vi "SYST_PRES.vi"(0 "VISA IN":refnum<visa-resource-name>, 5 "error in":errorcluster) -> (14 "VISA Out":refnum<visa-resource-name>, 19 "error out":errorcluster)   [LabVIEW 2018, in "PNA-X.lvlib"] (continued)
\n(Read-Write) Sets the type of the specified marker. \nSee Critical Note \nParameters \n<cnum> Channel number of the measurement. There must be a selected measurement \non that channel. If unspecified, <cnum> is set to 1. \n<mkr> Any marker number from 1 to 10; if unspecified, value is set to 1 \n<char> Choose from: \nNORMal - a marker that stays on the assigned X-axis position unless moved or \nsearching. \nFIXed - a marker that will not leave the assigned X or current Y-axis position. \nExamples CALC:MARK:TYPE NORM \ncalculate2:marker2:type fixed \nQuery Syntax CALCulate<cnum>:MARKer<mkr>:TYPE? \nReturn Type Character \n1540\n\nDefault NORMal \nCALCulate<cnum>:MARKer<mkr>:SET <char> \n(Write-only) Sets the selected instrument setting to assume the value of the specified marker. \nMarker Functions CENT, SPAN, STARt, and STOP do not work with channels that are in CW or \nSegment Sweep mode. \nSee Critical Note \nParameters \n<cnum> Channel number of the measurement. There must be a selected measurement \non that channel. If unspecified, <cnum> is set to 1. \n<mkr> Any marker number from 1 to 10; if unspecified, value is set to 1 \n<char> Choose from: \nCENTer - changes center frequency to the value of the marker \nSPAN - changes the sweep span to the span that is defined by the delta marker \nand the marker that it references. Unavailable if there is no delta marker. \nSTARt - changes the start frequency to the value of the marker \nSTOP - changes the stop frequency to the value of the marker \nRLEVel - changes the reference level to the value of the marker \nDELay - changes the line length at the receiver input to the phase slope at the \nactive marker stimulus position. \nExamples CALC:MARK:SET CENT \ncalculate2:marker8:set span \nQuery Syntax Not Applicable \nDefault Not Applicable \nCALCulate<cnum>:MARKer<mkr>[:STATe] <ON|OFF> \n1541\n\n(Read-Write) Turns the specified marker ON or OFF. Marker 10 is the Reference Marker. To turn \nall markers off, use CALC:MARK:AOFF. \nSee Critical Note \nParameters \n<cnum> Channel number of the measurement. There must be a selected measurement \non that channel. If unspecified, <cnum> is set to 1. \n<mkr> Any marker number from 1 to 10; if unspecified, value is set to 1. \n<ON|OFF> ON (or 1) - turns marker ON. \nOFF (or 0) - turns marker OFF. \nExamples CALC:MARK ON \ncalculate2:marker8 on \nQuery Syntax CALCulate<cnum>:MARKer<mkr>:STATe? \nReturn Type Boolean (1 = ON, 0 = OFF) \nDefault Off \nCALCulate<cnum>:MARKer<mkr>:X <num> \n(Read-Write) Sets the marker's X-axis value (frequency, power, or time). If the marker is set as delta, \nthe SET and QUERY data is relative to the reference marker. \nSee Critical Note \nParameters \n<cnum> Channel number of the measurement. There must be a selected measurement \non that channel. If unspecified, <cnum> is set to 1. \n<mkr> Any marker number from 1 to 10; if unspecified, value is set to 1. \n<num> Any X-axis position within the measurement span of the marker. \nNote: This command will accept MIN or MAX instead of a numeric \nparameter. See SCPI Syntax for more information. \nExamples CALC:MARK:X 100Mhz \ncalculate2:marker8:x maximum \nQuery Syntax CALCulate<cnum>:MARKer<mkr>:X? \nReturn Type Numeric \nDefault First Marker turns ON in the middle of the X-axis span. Subsequent markers \nturn ON at the position of the active marker. \n1542\n\nCALCulate<cnum>:MARKer<mkr>:Y? \n(Read-only) Reads the marker's Y-axis value. The format of the value depends on the current \nCALC:MARKER:FORMAT setting. If the marker is set as delta, the data is relative to the reference \nmarker. The query always returns two numbers: \nSmith and Polar formats - (Real, Imaginary) \nLINPhase and LOGPhase - (Real, Imaginary) \nAll other formats - (Value,0) \nNote: To accurately read the marker Y-axis value with trace smoothing applied, the requested format \nmust match the displayed format. Otherwise, the returned value is un-smoothed data. For example, to \nread the smoothed marker value when measuring group delay, both the display format and the marker \nformat must be set to (Group) Delay. \nSee Critical Note \nParameters \n<cnum> Channel number of the measurement. There must be a selected measurement \non that channel. If unspecified, <cnum> is set to 1. \n<mkr> Any marker number from 1 to 10; if unspecified, value is set to 1. \nExamples CALC:MARK:Y? \ncalculate2:marker3:y? \nQuery Syntax CALCulate<cnum>:MARKer<mkr>:Y? \nReturn Type Numeric \nDefault Not applicable \nLast modified: \nMarch 27, 2007 Corrected Set? \nDec. 4, 2006 Added smoothing note to Y? \n1543\n\nCalculate:Math Commands \nControls math operations on the currently selected measurement and memory. \nClick on a blue keyword to view the command details. \nSee Also \nExample Programs \nLearn about Math Operations \nSynchronizing the PNA and Controller \nSCPI Command Tree \nCritical Note: CALCulate commands act on the selected measurement. You can select one \nmeasurement for each channel using Calc:Par:Select \nCALCulate<cnum>:MATH:FUNCtion <char> \n(Read-Write) Sets math operations on the currently selected measurement and the trace stored in \nmemory. (There MUST be a trace stored in Memory. See CALC:MATH MEM) \nSee Critical Note \nParameters \n<cnum> Channel number of the measurement. There must be a selected measurement \non that channel. If unspecified, <cnum> is set to 1. \n<char> The math operation to be applied. Choose from the following: \nNORMal Trace data only \nADD Data + Memory \nSUBTract Data - Memory \nMULTiply Data * Memory \nDIVide Data / Memory \n1544\n\nExamples CALC:MATH:FUNC NORM \ncalculate2:math:function subtract \nQuery Syntax CALCulate<cnum>:MATH:FUNCtion? \nReturn Type Character \nDefault NORMal \nCALCulate<cnum>:MATH:MEMorize \n(Write-only) Puts the currently selected measurement trace into memory. (Data-> Memory). \nSee Critical Note \nParameters \n<cnum> Channel number of the measurement. There must be a selected measurement \non that channel. If unspecified, <cnum> is set to 1. \nExamples CALC:MATH:MEM \ncalculate2:math:memorize \nQuery Syntax Not applicable \nDefault Not applicable \n1545\n\nCalculate:Mixer Command \nCALCulate<ch>:MIXer:XAXis <char> \n(Read-Write) Sets or returns the swept parameter to display on the X-axis for the selected FCA \nmeasurement. Learn more about X-axis display. \nCritical Note: CALCulate commands act on the selected measurement. You can select one \nmeasurement for each channel using Calc:Par:Select \nParameters \n<ch> Any existing channel number. If unspecified, value is set to 1. \n<char> Parameter to display on the X-axis. Choose from: \nINPUT - Input frequency span \nOUTPUT - Output frequency span \nLO_1 - First LO frequency span \nLO_2 - Second LO frequency span \nExamples CALC:MIX:XAX INPUT \ncalc2:mixer:xaxis output \nSee an example that creates, selects, and calibrates an SMC and \nVMC measurement using SCPI. \nQuery Syntax CALCulate<ch>:MIXer:XAXis? \nReturn Type Character \nDefault OUTPUT \n1546\n\nCalculate:Normalize Commands \nSpecifies the normalization features used for a receiver power calibration. \nThese commands are Superseded (Sept 2004). \nSee the replacement commands in a new Receiver Power Cal example. \nClick on a blue keyword to view the command details. \nSee Also \nExample Programs \nLearn about Receiver Cal \nSCPI Command Tree \nSave and recall your receiver power calibration (which use .CST file commands): \nSENS:CORR:CSET:SAVE \nSENS:CORR:CSET[:SEL] \nOr use these two commands and specify either .STA or .CST file extensions: \nMMEM:LOAD \nMMEM:STOR \nCritical Note: CALCulate commands act on the selected measurement. You can select one \nmeasurement for each channel using Calc:Par:Select \nCALCulate<cnum>:NORMalize[:IMMediate] Superseded \n1547\n\nNote: This command is replaced with SENS:CORR:COLL:METH RPOWer and \nSENS:CORR:COLL[:ACQ] POWer \nSee an example of a Receiver Power Calibration. \n(Write only) Stores the selected measurement�s data to that measurement�s �divisor� buffer for use by \nthe Normalization data processing algorithm. This command is not compatible with ratioed \nmeasurements such as S-parameters. It is intended for receiver power calibration when the selected \nmeasurement is of an unratioed power type. \nSee Critical Note \nParameters \n<cnum> Channel number of the measurement. There must be a selected measurement \non that channel. If unspecified, <cnum> is set to 1. \nExamples CALC:NORM \ncalculate1:normalize:immediate \nQuery Syntax Not Applicable \nDefault Not Applicable \nCALCulate<cnum>:NORMalize:STATe <ON | OFF> Superseded \nNote: This command is replaced with SENS:CORR[:STATe] ON|OFF \n(Read-Write) Specifies whether or not normalization is applied to the measurement. Normalization is \nenabled only for measurements of unratioed power where it serves as a receiver power calibration. \nSee Critical Note \nParameters \n<cnum> Channel number of the measurement. There must be a selected measurement \non that channel. If unspecified, <cnum> is set to 1. \n<ON | OFF> ON (or 1) - normalization is applied to the measurement. \nOFF (or 0) � normalization is NOT applied to the measurement. \nExamples CALC:NORM:STAT ON \ncalculate2:normalize:state off \nQuery Syntax CALCulate<cnum>:NORMalize:STATe? \nReturn Type Boolean (1 = ON, 0 = OFF) \nDefault OFF \n1548\n\nCALCulate<cnum>:NORMalize:INTerpolate[:STATe] <ON | OFF> Superseded \nNote: This command is replaced with SENS:CORR:INT[:STATe] ON|OFF \n(Read-Write) Turns normalization interpolation ON or OFF. Normalization is enabled only for \nmeasurements of unratioed power, where it serves as a receiver power calibration. \nSee Critical Note \nParameters \n<cnum> Channel number of the measurement. There must be a selected measurement \non that channel. If unspecified, <cnum> is set to 1. \n<ON | OFF> ON (or 1) � turns interpolation ON. \nOFF (or 0) � turns interpolation OFF. \nExamples CALC:NORM:INT ON \ncalculate2:normalize:interpolate:state off \nQuery Syntax CALCulate<cnum>:NORMalize:INTerpolate[:STATe]? \nReturn Type Boolean (1 = ON, 0 = OFF) \nDefault ON \n1549\n\nCalculate:Offset Commands \nAllows the data trace magnitude and phase to be offset. \nClick on a blue keyword to view the command details. \nSee Also \nExample Programs \nLearn about Magnitude Offset \nLearn about Phase Offset \nSynchronizing the PNA and Controller \nSCPI Command Tree \nCritical Note: CALCulate commands act on the selected measurement. You can select one \nmeasurement for each channel using Calc:Par:Select \nCALCulate<cnum>:OFFSet:MAGNitude <num>\n1550\n\n(Read-Write) Offsets the data trace magnitude by the specified value. \nTo offset the data trace magnitude to a slope value that changes with frequency, use \nCALC:OFFS:MAGN:SLOP \nSee Critical Note \nParameters \n<cnum> Channel number of the measurement. There must be a selected measurement \non that channel. If unspecified, <cnum> is set to 1. \n<num> Offset value in dB. \nExamples CALC:OFFS:MAGN:4 \ncalculate1:offset:magnitude -2 \nQuery Syntax CALCulate<cnum>:OFFSet:MAGNitude? \nReturn Type Numeric \nDefault 0 \nCALCulate<cnum>:OFFSet:MAGNitude:SLOPe <num> \n(Read-Write) Offsets the data trace magnitude to a value that changes linearly with frequency. The \noffset slope begins at 0 Hz. \nSee Critical Note \nParameters \n<cnum> Channel number of the measurement. There must be a selected measurement \non that channel. If unspecified, <cnum> is set to 1. \n<num> Offset slope value in dB/ 1GHz. \nExamples CALC:OFFS:MAGN:SLOP 1 'Offset slope set to 1dB/GHz \ncalculate1:offset:magnitude:slope -2 'Offset slope set to - \n2dB/GHz \nQuery Syntax CALCulate<cnum>:OFFSet:MAGNitude:SLOPe? \nReturn Type Numeric \nDefault 0 \nCALCulate<cnum>:OFFSet:PHASe <num>[<char>] \n1551\n\n(Read-Write) Sets the phase offset for the selected measurement. \nSee Critical Note \nParameters \n<cnum> Channel number of the measurement. There must be a selected measurement \non that channel. If unspecified, <cnum> is set to 1. \n<num> Offset phase value. Choose any number between: \n-360 and 360 \n<char> Units for phase. OPTIONAL. Choose either: \nDEG - Degrees (default) \nRAD - Radians \nExamples CALC:OFFS:PHAS 10 \ncalculate:offset:phase 20rad \nQuery Syntax CALCulate:OFFSet:PHASe? \nReturn Type Numeric, returned value always in degrees \nDefault 0 degrees \n1552\n\nCalculate:Parameter Commands \nLists, creates, selects and deletes measurements. \nClick on a blue keyword to view the command details. \nSee Also \nExample Programs \nLearn about Measurement Parameters \nSynchronizing the PNA and Controller \nSCPI Command Tree \nCritical Note: CALCulate commands act on the selected measurement. You can select one \nmeasurement for each channel using Calc:Par:Select \nCALCulate<cnum>:PARameter:CATalog? \n(Read-only) Returns the names and parameters of existing measurements for the specified channel. \nNote: For Balanced Measurements: CALC:PAR:CAT? may have an unexpected behavior. Learn \nmore. \nSee Critical Note \nParameters \n<cnum> Channel number of the measurements to be listed. If unspecified, <cnum> is \nset to 1. \nExamples CALC:PAR:CAT? \ncalculate2:parameter:catalog? \nReturn Type String - \"<measurement name>,<parameter>,[<measurement \nname>,<parameter>...]\" \n1553\n\nDefault \"CH1_S11_1,S11\" \nCALCulate<cnum>:PARameter:DEFine <Mname>,<param>[,port] Superseded \nNote: This command is replaced with CALC:PAR:DEFine:EXTended. This command will continue \nto work for up to 4 port parameters. \n(Write-only) Creates a measurement but does NOT display it. \nThere is no limit to the number of measurements that can be created. However, there is a limit to the \nnumber of measurements that can be displayed. See Traces, Channels, and Windows on the PNA. \nUse DISP:WIND:STATe to create a window if it doesn't already exist. \nUse DISP:WIND<wnum>:TRAC<tnum>:FEED <Mname> to display the measurement. \nFor FCA Measurements see CALC:CUST:DEF \nYou must select the measurement (CALC<cnum>:PAR:SEL <mname>) before making additional \nsettings. \nSee Critical Note \nParameters \n<cnum> Channel number of the new measurement. If unspecified, value is set to 1. \n<Mname> Name of the measurement. Any non-empty, unique string, enclosed in quotes. \n<param> \nFor S-parameters: \nAny S-parameter available in the PNA \nFor ratioed measurements: \nAny two receivers that are available in the PNA. (See the block diagram \nshowing the receivers in YOUR PNA.) \nFor example: AR1 (this means A/R1) \nFor non-ratioed measurements: \nAny receiver that is available in the PNA. (See the block diagram showing \nthe receivers in YOUR PNA.) \nFor example: A \n1554\n\nFor Balanced Measurements: \nFirst create an S-parameter measurement, then change the measurement \nusing CALC:FSIM:BAL commands. See an example. \nFor FCA Measurements see CALC:CUST:DEF \n[port] Optional argument; \nFor multi-port reflection S-parameter measurements: specifies the PNA port \nwhich will provide the load for the calibration. This argument is ignored if a \ntransmission S-parameter is specified. \nFor all non S-parameter measurements: specifies the source port for the \nmeasurement. \nExamples CALC4:PAR:DEF 'ch4_S33',S33,2 'Defines an S33 measurement with a \nload on port2 of the analyzer. \ncalculate2:parameter:define 'ch1_a', a, 1 'unratioed meas \ncalculate2:parameter:define 'ch1_a', ar1,1 'ratioed meas \nQuery Syntax Not Applicable; see Calc:Par:Cat? \nDefault Not Applicable \nCALCulate<cnum>:PARameter:DEFine:EXTended <Mname>,<param> \nNote: This command replaces CALC:PAR:DEF as it allows the creating of measurements using \nexternal multiport testsets. \n(Write-only) Creates a measurement but does NOT display it. \nThere is no limit to the number of measurements that can be created. However, there is a limit to the \nnumber of measurements that can be displayed. See Traces, Channels, and Windows on the PNA. \nUse DISP:WIND:STATe to create a window if it doesn't already exist. \nUse DISP:WIND<wnum>:TRAC<tnum>:FEED <Mname> to display the measurement. \nYou must select the measurement (CALC<cnum>:PAR:SEL <mname>) before making additional \nsettings. \nSee Critical Note \nParameters \n1555\n\n<cnum> Channel number of the new measurement. If unspecified, value is set to 1. \n<Mname> (String) Name of the measurement. Any non-empty, unique string, enclosed in \nquotes. \n<param> \n(String ) Measurement Parameter to create. Case sensitive. \nFor S-parameters: \nAny S-parameter available in the PNA \nSingle-digit port numbers CAN be separated by \"_\" (underscore). For \nexample: \"S21\" or \"S2_1\" \nDouble-digit port numbers MUST be separated by underscore. For \nexample: \"S10_1\" \nFor ratioed measurements: \nAny two PNA physical receivers separated by forward slash '/' followed by \ncomma and source port. \nFor example: \"A/R1, 3\" \nLearn more about ratioed measurements \nSee a block diagram showing the receivers in YOUR PNA. \nFor non-ratioed measurements: \nAny PNA physical receiver followed by comma and source port. \nFor example: \"A, 4\" \nLearn more about unratioed measurements. \nSee the block diagram showing the receivers in YOUR PNA. \nWith PNA Rev 6.2, Ratioed and Unratioed measurements can also use logical \nreceiver notation to refer to receivers. This notation makes it easy to refer to \nreceivers with an external test set connected to the PNA. You do not need to \nknow which physical receiver is used for each test port. Learn more. \nFor ADC measurements: \nAny ADC receiver in the PNA followed by a comma, then the source port. \nFor example: \"AI1,2\" indicates the Analog Input1 with source port of 2. \n1556\n\nLearn more about ADC receiver measurements. \nFor Balanced Measurements: \nFirst create an S-parameter measurement, then change the measurement \nusing CALC:FSIM:BAL \"define\" commands. See an example. \nExamples CALC4:PAR:DEF:EXT 'ch4_S33', 'S33' 'Defines an S33 measurement \ncalculate2:parameter:define:extended 'ch1_a', 'b9, 1' 'logical \nreceiver notation for unratioed meas of test port 9 receiver with \nsource port 1. \ncalculate2:parameter:define:extended 'ch1_a', 'b9/a10,1' 'logical \nreceiver notation for ratioed meas of test port 9 receiver divided \nby the reference receiver for port 10 using source port 1 \nQuery Syntax Not Applicable; see Calc:Par:Cat? \nDefault Not Applicable \nCALCulate<cnum>:PARameter:DELete[:NAME] <Mname> \n(Write-only) Deletes the specified measurement. \nSee Critical Note \nParameters \n<cnum> Channel number of the measurement. There must be a selected measurement \non that channel. If unspecified, <cnum> is set to 1. \n<Mname> String - Name of the measurement \nExamples CALC:PAR:DEL 'TEST' \ncalculate2:parameter:delete 'test' \nQuery Syntax Not Applicable \nDefault Not Applicable \nCALCulate:PARameter:DELete:ALL \n1557\n\n(Write-only) Deletes all measurements on the PNA. \nSee Critical Note \nParameters \nExamples CALC:PAR:DEL:ALL \nQuery Syntax Not Applicable \nDefault Not Applicable \nCALCulate<cnum>:PARameter:MNUMber? \n(Read-only) Returns the measurement number of the selected measurement. This is useful when \nneeding to identify a measurement by number, such as with Status:Ques:Lim or Status:Oper:Aver \ncommands. \nSee Critical Note \nParameters \n<cnum> Channel number of the measurement. If unspecified, <cnum> is set to 1. \nExamples CALC:PAR:MNUM? \ncalculate2:parameter:mnumber? \nReturn Type Numeric \nDefault Not Applicable \nCALCulate<cnum>:PARameter:MODify <param> Superseded \nNote: This command is replaced with CALC:PAR:MOD:EXT. This command will continue to work \nfor up to 4 port parameters. \n(Write-only) Modifies a standard measurement using the same arguments as CALC:PAR:DEF. To \nmodify an FCA measurement, use CALC:CUST:MOD. \nSee Critical Note \nParameters \n<cnum> Channel number of the measurement. The selected measurement on that \nchannel will be changed. If unspecified, <cnum> is set to 1. \n<param> Measurement parameter to change to. Use the same <param> arguments as \nCALC:PAR:DEF. \nExamples SYST:PRESET \n1558\n\nCALC:PAR:DEF \"MyMeas\", S11 \nCALC:PAR:SEL \"MyMeas\" \nCALC:PAR:MOD AR1 'changes the selected S11 measurement to an A/R1 \nmeasurement \nQuery Syntax Not Applicable \nDefault Not Applicable \nCALCulate<cnum>:PARameter:MODify:EXTended <param> \nNote: This command replaces CALC:PAR:MOD as it allows modification of measurements using \nexternal multiport testsets. \n(Write-only) Modifies a standard measurement using the same arguments as CALC:PAR:DEF:EXT. \nTo modify an FCA measurement, use CALC:CUST:MOD. \nSee Critical Note \nParameters \n<cnum> Channel number of the measurement. The selected measurement on that \nchannel will be changed. If unspecified, <cnum> is set to 1. \n<param> (String) New measurement parameter. Use the same <param> arguments as \nCALC:PAR:DEF:EXT. \nExamples SYST:PRESET \nCALC:PAR:DEF:EXT \"MyMeas\", \"S10_1\" \nCALC:PAR:SEL \"MyMeas\" \nCALC:PAR:MOD:EXT \"a4b4,1\" 'changes the selected S10_1 \nmeasurement to an a4/b4 measurement with source port 1 \nQuery Syntax Not Applicable \nDefault Not Applicable \nCALCulate<cnum>:PARameter:SELect <Mname> \n1559\n\n(Read-Write) Sets the selected measurement. Most CALC: commands require that this command be \nsent before a setting change is made. One measurement on each channel can be selected at the same \ntime. To obtain a list of currently named measurements, use CALC:PAR:CAT? \nParameters \n<cnum> Channel number of the measurement to be selected. If unspecified, <cnum> is \nset to 1. \n<Mname> String - Name of the measurement. (Do NOT include the parameter name.) \nExamples CALC:PAR:SEL 'TEST' \ncalculate2:parameter:select 'test' \nQuery Syntax CALCulate:PARameter:SELect? \nReturn Type String \nDefault The preset measurement name is \"CH1_S11_1\" \nLast modified: \nApril 19, 2007 MX Added ADC meas \n9/12/06 MQ New Extended commands. \n1560\n\nCalculate:RData? Command \nCritical Note: CALCulate commands act on the selected measurement. You can select one \nmeasurement for each channel using Calc:Par:Select \nCALCulate<cnum>:RDATA? <char> \n(Read-only) Returns receiver data for the selected measurement. To query measurement data, see \nCALC:DATA? \nParameters \n<cnum> Channel number of the measurement. There must be a selected measurement \non that channel. If unspecified, <cnum> is set to 1. \n<char> Choose from any physical receiver in the PNA. \nFor example: \"A\" \nAlso, REF - returns data for either R1 or R2 data depending on the source port \nof the selected measurement. \nSee the block diagram showing the receivers in YOUR PNA. \nNote: Logical receiver notation is NOT allowed with this command. Learn \nmore. \nExample GPIB.Write \"INITiate:CONTinuous OFF\" \nGPIB.Write \"INITiate:IMMediate;*wai\" \nGPIB.Write \"CALCulate:RDATA? A\" \nGPIB.Write \"CALCulate:RDATA? REF\" \nReturn Type Depends on FORM:DATA - Two numbers per data point \nDefault Not Applicable \nNotes: \nGenerally when you query the analyzer for data, you expect that the number of data values returned will \nbe consistent with the number of points in the sweep. \nHowever, if you query receiver data while the instrument is sweeping, the returned values may contain \nzeros. For example, if your request for receiver data is handled on the 45th point of a 201 point sweep, \nthe first 45 values will be valid data, and the remainder will contain complex zero. \nThis can be avoided by synchronizing this request with the end of a sweep or putting the channel in \nhold mode. \n1561\n\nLearn about Unratioed Measurements \n1562\n\nCalculate:Smoothing Commands \nControls point-to-point smoothing. Smoothing is a noise reduction technique that averages adjacent \ndata points in a measurement trace. Choose the amount of smoothing by specifying either the number \nof points or the aperture. Smoothing is not the same as CALC:AVERage which averages each data \npoint over a number of sweeps. \nClick on a blue keyword to view the command details. \nSee Also \nExample Programs \nLearn about Smoothing \nSynchronizing the PNA and Controller \nSCPI Command Tree \nCritical Note: CALCulate commands act on the selected measurement. You can select one \nmeasurement for each channel using Calc:Par:Select \nCALCulate<cnum>:SMOothing:APERture <num> \n(Read-Write) Sets the amount of smoothing as a percentage of the number of data points in the \nchannel. \nSee Critical Note \nParameters \n<cnum> Channel number of the measurement. There must be a selected measurement \non that channel. If unspecified, <cnum> is set to 1. \n<num> Percentage value. Choose any number between: \n1 and 25 \nExamples CALC:SMO:APER 2 \ncalculate2:smoothing:aperture 20.7 \nQuery Syntax CALCulate<cnum>:SMOothing:APERture? \nReturn Type Numeric \n1563\n\nDefault 1.5 \nCALCulate<cnum>:SMOothing:POINts <num> \n(Read-Write) Sets the number of adjacent data points to average. \nSee Critical Note \nParameters \n<cnum> Channel number of the measurement. There must be a selected measurement \non that channel. If unspecified, <cnum> is set to 1. \n<num> Number of points from 1 point to maximum of 25% of data points in the \nchannel. For example: if number of points in a data trace = 401, the maximum \nvalue for points = 100. The points value is always rounded to the closest odd \nnumber. \nExamples CALC:SMO:POIN 50 \ncalculate2:smoothing:points 21 \nQuery Syntax CALCulate<cnum>:SMOothing:POINts? \nReturn Type Numeric \nDefault 3 \nCALCulate<cnum>:SMOothing[:STATe] <ON | OFF> \n(Read-Write) Turns data smoothing ON or OFF. \nSee Critical Note \nParameters \n<cnum> Channel number of the measurement. There must be a selected measurement \non that channel. If unspecified, <cnum> is set to 1. \n<ON | OFF> ON (or 1) - turns smoothing ON. \nOFF (or 0) - turns smoothing OFF. \nExamples CALC:SMO ON \ncalculate2:smoothing:state off \nQuery Syntax CALCulate<cnum>:SMOothing[:STATe]? \nReturn Type Boolean (1 = ON, 0 = OFF) \nDefault OFF \n1564\n\n1565\n\nCalculate:Transform Commands \nSpecifies the settings for time domain transform. \nClick on a blue keyword to view the command details. \nSee Also \nExample Programs \nLearn about Time Domain \nSynchronizing the PNA and Controller \nSCPI Command Tree \nCritical Note: CALCulate commands act on the selected measurement. You can select one \nmeasurement for each channel using Calc:Par:Select \nCALCulate<cnum>:TRANsform:COUPle:PARameters <num> \n(Read-Write) Specifies the time domain transform parameters to be coupled. The settings for those \nparameters will be copied from the selected measurement to all other measurements on the channel. \nTo turn coupling ON and OFF, use SENS:COUP:PAR \nTo specify Gating parameters to couple, use CALC:FILT:COUP:PAR \nLearn more about Time Domain Trace Coupling \nSee Critical Note \nParameters \n<cnum> Channel number of the measurement. There must be a selected measurement \non that channel. If unspecified, <cnum> is set to 1. \n<num> (Numeric) Parameters to couple. To specify more than one parameter, add the \n1566\n\nnumbers. \n1 - Transform Stimulus (Start, Stop, Center, and Span TIME settings.) \n2 - Transform State (ON / OFF) \n4 - Transform Window (Kaiser Beta / Impulse Width) \n8 - Transform Mode (Low Pass Impulse, Low Pass Step, Band Pass) \n16 - Transform Distance Marker Units \nExamples 'To couple all parameters: \nCALC:TRAN:COUP:PAR 31 \n'To couple Stimulus and Mode: \ncalculate2:transform:couple:parameters 9 \nQuery Syntax CALCulate<cnum>:TRANsform:COUPle:PARameters? \nReturn Type Numeric \nDefault 29 (All parameters except 2 - Transform State) \nCALCulate<cnum>:TRANsform:TIME:CENTer <num> \n(Read-Write) Sets the center time for time domain measurements. \nSee Critical Note \nParameters \n<cnum> Channel number of the measurement. There must be a selected measurement \non that channel. If unspecified, <cnum> is set to 1. \n<num> Center time in seconds; any number between: \n� (number of points-1) / frequency span \nNote: This command will accept MIN or MAX instead of a numeric \nparameter. See SCPI Syntax for more information. \nExamples CALC:TRAN:TIME:CENT 1e-8 \ncalculate2:transform:time:center 15 ps \nQuery Syntax CALCulate<cnum>:TRANsform:TIME:CENTer? \nReturn Type Numeric \nDefault 0 \n1567\n\nCALCulate<cnum>:TRANsform:TIME:IMPulse:WIDTh <num> \n(Read-Write) Sets the impulse width for the transform window. \nSee Critical Note \nParameters \n<cnum> Channel number of the measurement. There must be a selected measurement \non that channel. If unspecified, <cnum> is set to 1. \n<num> Impulse width in seconds; Choose any number between: \n.6 / frequency span and 1.39 / frequency span \nExamples CALC:TRAN:TIME:IMP:WIDTh 10 \ncalculate2:transform:time:impulse:width 13 \nQuery Syntax CALCulate<cnum>:TRANsform:TIME:IMPulse:WIDTh? \nReturn Type Numeric \nDefault .98 / Default Span \nCALCulate<cnum>:TRANsform:TIME:KBESsel <num> \n(Read-Write) Sets the parametric window for the Kaiser Bessel window. \nSee Critical Note \nParameters \n<cnum> Channel number of the measurement. There must be a selected measurement \non that channel. If unspecified, <cnum> is set to 1. \n<num> Window width for Kaiser Bessel in seconds; Choose any number between: \n0.0 and 13.0 \nExamples CALC:TRAN:TIME:KBES 10 \ncalculate2:transform:time:kbessel 13 \nQuery Syntax CALCulate<cnum>:TRANsform:TIME:KBESsel? \nReturn Type Numeric \nDefault 6 \nCALCulate<cnum>:TRANsform:TIME:LPFREQuency \n1568\n\n(Write-only) Sets the start frequencies in LowPass Mode. \nSee Critical Note \nParameters \n<cnum> Channel number of the measurement. There must be a selected measurement \non that channel. If unspecified, <cnum> is set to 1. \nExamples CALC:TRAN:TIME:LPFR \ncalculate2:transform:time:lpfrequency \nQuery Syntax Not applicable \nDefault Not applicable \nCALCulate<cnum>:TRANsform:TIME:MARKer:MODE <char> \n(Read-Write) Specifies the measurement type in order to determine the correct marker distance. \nSelect Auto for S-Parameter measurements. \nSelect Reflection or Transmission for arbitrary ratio or unratioed measurements. \nThis setting affects the display of ALL markers for only the ACTIVE measurement. \nLearn more about Distance Markers. \nSee Critical Note \nParameters \n<cnum> Channel number of the measurement. There must be a selected measurement \non that channel. If unspecified, <cnum> is set to 1. \n<char> Choose from: \nAUTO If the active measurement is an S-Parameter, automatically chooses \nreflection or transmission. If non S-Parameter measurements, reflection is \nchosen. \nREFLection Displays the distance from the source to the receiver divided by \ntwo (to compensate for the return trip.) \nTRANsmission Displays the distance from the source to the receiver. \nExamples CALC:TRAN:TIME:MARK:MODE REFL \ncalculate2:transform:time:marker:mode auto \nQuery Syntax CALCulate<cnum>:TRANsform:TIME:MARKer:MODE? \n1569\n\nReturn Type Character \nDefault Auto \nCALCulate<cnum>:TRANsform:TIME:MARKer:UNIT <char> \n(Read-Write) Specifies the unit of measure for the display of marker distance values. This settings \naffects the display of ALL markers for only the ACTIVE measurement (unless Distance Maker Units \nare coupled using CALC:TRAN:COUP:PAR. \nLearn more about Distance Markers. \nSee Critical Note \nParameters \n<cnum> Channel number of the measurement. There must be a selected measurement \non that channel. If unspecified, <cnum> is set to 1. \n<char> Choose from: \nMETRs \nFEET \nINCHes \nExamples CALC:TRAN:TIME:MARK:UNIT INCH \ncalculate2:transform:time:marker:unit feet \nQuery Syntax CALCulate<cnum>:TRANsform:TIME:MARKer:UNIT? \nReturn Type Character \nDefault METRs \nCALCulate<cnum>:TRANsform:TIME:SPAN <num> \n1570\n\n(Read-Write) Sets the span time for time domain measurements. \nSee Critical Note \nParameters \n<cnum> Channel number of the measurement. There must be a selected measurement \non that channel. If unspecified, <cnum> is set to 1. \n<num> Span time in seconds; any number between: \n0 and 2* [(number of points-1) / frequency span] \nNote: This command will accept MIN or MAX instead of a numeric \nparameter. See SCPI Syntax for more information. \nExamples CALC:TRAN:TIME:SPAN 1e-8 \ncalculate2:transform:time:span maximum \nQuery Syntax CALCulate<cnum>:TRANsform:TIME:SPAN? \nReturn Type Numeric \nDefault 20 ns \nCALCulate<cnum>:TRANsform:TIME:STARt <num> \n(Read-Write) Sets the start time for time domain measurements. \nSee Critical Note \nParameters \n<cnum> Channel number of the measurement. There must be a selected measurement \non that channel. If unspecified, <cnum> is set to 1. \n<num> Start time in seconds; any number between: \n� (number of points-1) / frequency span \nNote: This command will accept MIN or MAX instead of a numeric \nparameter. See SCPI Syntax for more information. \nExamples CALC:TRAN:TIME:STAR 1e-8 \ncalculate2:transform:time:start minimum \nQuery Syntax CALCulate<cnum>:TRANsform:TIME:STARt? \nReturn Type Numeric \nDefault -10 ns \n1571\n\nCALCulate<cnum>:TRANsform:TIME:STATe <ON | OFF> \n(Read-Write) Turns the time domain transform capability ON or OFF. \nSee Critical Note \nNote: Sweep type must be set to Linear Frequency in order to use Time Domain Transform. \nParameters \n<cnum> Channel number of the measurement. There must be a selected measurement \non that channel. If unspecified, <cnum> is set to 1. \n<ON|OFF> ON (or 1) - turns time domain ON. \nOFF (or 0) - turns time domain OFF. \nExamples CALC:TRAN:TIME:STAT ON \ncalculate2:transform:time:state off \nQuery Syntax CALCulate<cnum>:TRANsform:TIME:STATe? \nReturn Type Boolean (1 = ON, 0 = OFF) \nDefault OFF \nCALCulate<cnum>:TRANsform:TIME:STOP <num> \n(Read-Write) Sets the stop time for time domain measurements. \nSee Critical Note \nParameters \n<cnum> Channel number of the measurement. There must be a selected measurement \non that channel. If unspecified, <cnum> is set to 1. \n<num> Stop time in seconds; any number between: \n� (number of points-1) / frequency span \nNote: This command will accept MIN or MAX instead of a numeric \nparameter. See SCPI Syntax for more information. \nExamples CALC:TRAN:TIME:STOP 1e-8 \ncalculate2:transform:time:stop maximum \nQuery Syntax CALCulate<cnum>:TRANsform:TIME:STOP? \nReturn Type Numeric \nDefault 10 ns \n1572\n\nCALCulate<cnum>:TRANsform:TIME:STEP:RTIMe <num> \n(Read-Write) Sets the step rise time for the transform window. \nSee Critical Note \nParameters \n<cnum> Channel number of the measurement. There must be a selected measurement \non that channel. If unspecified, <cnum> is set to 1. \n<num> Rise time in seconds; Choose any number between: \n.45 / frequency span and 1.48 / frequency span \nExamples CALC:TRAN:TIME:STEP:RTIM 1e-8 \ncalculate2:transform:time:step:rtime 15 ps \nQuery Syntax CALCulate<cnum>:TRANsform:TIME:STEP:RTIMe? \nReturn Type Numeric \nDefault .99 / Default Span \nCALCulate<cnum>:TRANsform:TIME:STIMulus <char> \n(Read-Write) Sets the type of simulated stimulus that will be incident on the DUT. \nSee Critical Note \nParameters \n<cnum> Channel number of the measurement. There must be a selected measurement \non that channel. If unspecified, <cnum> is set to 1. \n<char> Choose from: \nSTEP - simulates a step DUT stimulus \nIMPulse - simulates a pulse DUT stimulus \nSTEP can ONLY be used when CALC:TRAN:TIME:TYPE is set to LPASs \n(Lowpass). (STEP cannot be used with TYPE = BPASs.) \n:STIM STEP will set :TYPE to LPASs \n:TYPE BPASs will set :STIM to IMPulse \nExamples CALC:TRAN:TIME:STIM STEP \ncalculate2:transform:time:stimulus impulse \nQuery Syntax CALCulate<cnum>:TRANsform:TIME:STIMulus? \nReturn Type Character \n1573\n\nDefault IMPulse \nCALCulate<cnum>:TRANsform:TIME[:TYPE] <char> \n(Read-Write) Sets the type of time domain measurement. \nSee Critical Note \nParameters \n<cnum> Channel number of the measurement. There must be a selected measurement \non that channel. If unspecified, <cnum> is set to 1. \n<char> Type of measurement. Choose from: \nLPASs - Lowpass; Must also send CALC:TRAN:TIME:LPFRequency before \ncalibrating. \nBPASs - Bandpass; \nBPASs can only be used when CALC:TRAN:TIME:STIM is set to IMPulse. \n(BPASs cannot be used with :STIM = STEP) \n:STIM STEP will set :TYPE to LPASs \n:TYPE BPASs will set :STIM to IMPulse \nExamples CALC:TRAN:TIME LPAS \ncalculate2:transform:time:type bpas \nQuery Syntax CALCulate<cnum>:TRANsform:TIME[:TYPE]? \nReturn Type Character \nDefault BPAS \n1574\n\nControl Commands \nSpecifies the settings to remotely control the rear panel connectors and ECAL Module state. \nClick on a blue keyword to view the command details. \nRed command is superseded. \nSee Also \nExample Programs \nSynchronizing the PNA and Controller \nSCPI Command Tree \nSee a pinout and detailed description of the rear panel connectors: \nAuxilliary IO connector \nExternal Test Set IO connector \nMaterial Handler IO connector \nCONTrol:CHANnel:INTerface:CONTrol:CONFig:RECall <string> \n1575\n\n(Write-only) Recalls an Interface Control configuration file. Learn more about Interface Control. \nParameters \n<string> File name and extension (.xml) of the configuration file to recall. Files are typically stored \nin the default folder \"C:/Program Files/Agilent/Network Analyzer/Documents\". To recall \nfrom a different folder, specify the full path name. \nExamples CONT:CHAN:INT:CONT:CONF:REC 'MyConfigFile.xml' \ncontrol:channel:interface:control:config:recall 'C:/Program \nFiles/Agilent/Network Analyzer/Documents/MyFile.xml' \nQuery Syntax Not Applicable \nDefault Not Applicable \nCONTrol:CHANnel:INTerface:CONTrol[:STATe] <bool> \n(Read-Write) Enables and disables ALL Interface Control settings. To send data, the individual interfaces must \nalso be enabled. Learn more about Interface Control. \nParameters \n<bool> Boolean \nFalse (0) - Interface Control is disabled;NO control data is sent. \nTrue (1) - Interface Control is enabled. \nExamples CONT:CHAN:INT:CONT 1 \ncontrol:channel:interface:control:state 0 \nQuery Syntax CONTrol:CHANnel:INTerface:CONTrol[:STATe]? \nReturn Type Boolean \nDefault False (0) \nCONTrol:ECAL:MODule[num]:PATH:COUNt? <name> \n(Read-only) Returns the number of unique states that exist for the specified path name on the selected ECal \nmodule. \nThis command performs exactly the same function as SENS:CORR:CKIT:ECAL:PATH:COUNt? \nUse the CONT:ECAL:MOD:PATH:STAT command to set the module into one of those states. \nUse SENS:CORR:CKIT:ECAL:PATH:DATA? to read the data for a state. \n1576\n\nParameters \n[num] Optional argument. USB number of the ECal module. If unspecified (only one ECal \nmodule is connected to the USB), <num> is set to 1. If two or more modules are \nconnected, use SENS:CORR:CKIT:ECAL:LIST? to determine how many, and \nSENS:CORR:CKIT:ECAL:INF? to verify their identities. \n<name> Name of the path for which to read number of states. Choose from: \nReflection paths \nA\nB\nC (4-port modules) \nD (4-port modules) \nTransmission paths \nAB \nAC (4-port modules) \nAD (4-port modules) \nBC (4-port modules) \nBD (4-port modules) \nCD (4-port modules) \nNote: For each transmission path, the first of the available states is the through state, \nthe second is the confidence (attenuator) state. \nExamples CONT:ECAL:MOD:PATH:COUNt? A \ncontrol:ecal:module2:path:count? cd \nReturn Type Integer \nDefault Not Applicable \nCONTrol:ECAL:MODule[num]:PATH:STATe <path>, <stateNum> \n(Write-only) Sets the internal state of the selected ECAL module. This command supersedes \nCONT:ECAL:MOD:STAT. \n1577\n\nUse CONT:ECAL:MOD:PATH:COUN? to read the number of unique states that exist for the specified path \nname on the module. \nUse SENS:CORR:CKIT:ECAL:PATH:DATA? to read the data for a state (from the module memory) \ncorresponding to the stimulus values of a channel. \nParameters \n[num] Optional argument. USB number of the ECal module. If unspecified (only one ECal \nmodule is connected to the USB), <num> is set to 1. If two or more modules are \nconnected, use SENS:CORR:CKIT:ECAL:LIST? to determine how many, and \nSENS:CORR:CKIT:ECAL:INF? to verify their identities. \n<path> Path name for which to set a state. Choose from: \nReflection paths \nA\nB\nC (4-port modules) \nD (4-port modules) \nTransmission paths \nAB \nAC (4-port modules) \nAD (4-port modules) \nBC (4-port modules) \nBD (4-port modules) \nCD (4-port modules) \n<stateNum> Number of the state to set. Refer to the following table to associate the <stateNum> with \na state in your ECal module. \nIn addition, CONT:ECAL:MOD:PATH:COUNt? returns the number of states in the \nspecified ECal module. \n1578\n\n<stateNum> N4432A and \nN4433A \nStates \nN4431A \nStates \nN469x \nStates** \n8509x States \nOne-Port Reflection States \n1 Open Open Impedance 1 Open \n2 Short Short Impedance 2 Short \n3 Impedance 1 Impedance 1 Impedance 3 Impedance 1 \n4 Impedance 2 Impedance 2 Impedance 4 Impedance 2 \n5 Impedance 5 \n6 Impedance 6 \n7 Impedance 7 \nTwo-Port Transmission States \n1 Thru Thru Thru Thru \n2 Confidence Confidence Confidence Confidence \n** The following modules have only FOUR Impedance states (1, 2, 3, 4): N4690B \n,N4691B ,N4692A ,N4696B. \nExamples CONT:ECAL:MOD:PATH:STATe A,5 \ncontrol:ecal:module2:state BC,1 \nQuery Syntax Not Applicable \nDefault Not Applicable \nCONTrol:ECAL:MODule[num]:STATe <value> Superseded \nThis command is replaced with CONT:ECAL:MOD:PATH:STATe. \n(Write-only) Sets the internal state of the selected ECAL module. \nParameters \n[num] Optional argument. USB number of the ECal module. If unspecified (only one ECal \nmodule is connected to the USB), <num> is set to 1. If two or more modules are \nconnected, use SENS:CORR:COLL:CKIT:INF? to verify their identity. \n1579\n\n<value> Integer code for switching the module. The following are codes for Agilent ECal \nmodules. \nAgilent 8509x Modules \nState Port A Port B \nOpen 0 0 \nShort 43 43 \nLoad 33 33 \nMismatch 4 16 \nThru 84 \nConfidence 20 \nAgilent N469x Modules \nState Port A Port B \nOpen 36 33 \nShort 39 45 \nLoad 37 37 \nMismatch \n(Offset short) \n53 53 \nImpedance 5 \n(Offset open) \n5 5 \nImpedance 6 \n(Offset short) \n21 21 \nImpedance 7 \n(Offset short) \n38 41 \nThru 42 \nConfidence 40 \n1580\n\nAgilent N4431A Modules \nState Port A Port B Port C Port D \nOpen -1398 -1384 -2774 -2654 \nShort -1350 -1381 -2582 -2642 \nLoad 26985 -26986 -26986 26985 \nMismatch -26986 26985 26985 -26986 \nPath Thru Confidence \nAB Path -2590 -598 \nAC Path -4011 85 \nAD Path -2517 16042 \nBC Path -1650 -598 \nBD Path -4011 85 \nCD Path -1352 16042 \nAgilent N4432A and N4433A Modules \nState Port A Port B Port C Port D \nOpen -6971 -11835 -14895 -14876 \nShort -14395 -12859 -14899 -14905 \nLoad -14907 -14907 -14907 -14907 \nOffset Short -9787 -6459 -14874 -14887 \n1581\n\nPath Thru Confidence \nAB Path 13765 30069 \nAC Path -10519 -2327 \nAD Path -10538 -2346 \nBC Path -5655 -1559 \nBD Path -5674 -1578 \nCD Path -15051 30069 \nExamples CONT:ECAL:MOD:STAT 36 \ncontrol:ecal:module2:state 38 \nQuery Syntax Not Applicable \nDefault Not Applicable \nCONTrol:SIGNal <conn>,<char> \n(Read-Write) Configures external triggering in the PNA. \nTrigger:Sequence:Source is automatically set to External when CONTrol:SIGNal is sent. \nEdge triggering is only available on some Microwave PNA models. \nFor more information, see External Triggering in the PNA. \nParameters \n<conn> Rear Panel connector to send or receive trigger signals. Choose from: \nBNC1 Trigger IN from rear-panel Trigger IN BNC connector \nAUXT Trigger IN from AUX IO connector Pin 19 \nNote: Only one of the input connectors is active at a time. When a command is sent to \none, the PNA automatically makes the other INACTIVE. \nBNC2 Trigger OUT to rear-panel Trigger OUT BNC connector. \nMATHtrigger - Trigger IN from rear-panel Material Handler connector Pin 18 \n<char> INACTIVE - Disables the specified connector <conn>. \nChoose from ONLY the following when <conn> is set to BNC1 or AUXT or \nMATHtrigger: \nTIENEGATIVE - (Trigger In Edge Negative) - Triggers the PNA when receiving a \nnegative going signal \n1582\n\nTIEPOSITIVE - (Trigger In Edge Positive) - Triggers the PNA when receiving a positive \ngoing signal \nTILLOW - (Trigger In Level Low) - Triggers the PNA when receiving a low level signal \nTILHIGH - (Trigger In Level High) - Triggers the PNA when receiving a High-level signal \nChoose from ONLY the following when <conn> is set to BNC2: \nUse CONTrol:SIGNal:TRIGger:OUTP to enable the BNC2 output. \nThe following selections send a positive or negative pulse before or after each trigger \nacquisition. This normally occurs each sweep unless a channel is in point trigger mode. \nTOPPAFTER - (Trigger Out Pulse Positive After) - Sends a POSITIVE going TTL pulse \nat the END of each trigger acquisition. \nTOPPBEFORE - (Trigger Out Pulse Positive Before) - Sends a POSITIVE going TTL \npulse at the START of each trigger acquisition. \nTOPNAFTER - (Trigger Out Pulse Negative After) - Sends a NEGATIVE going TTL \npulse at the END of each trigger acquisition. \nTOPNBEFORE - (Trigger Out Pulse Negative Before) - Sends a NEGATIVE going TTL \npulse at the START of each trigger acquisition. \nExamples CONT:SIGN BNC1,TIENEGATIVE \ncontrol:signal bnc2,toppbefore \nQuery Syntax CONTrol:SIGNal? <conn> \nIn addition to the arguments listed above, the following is also a possible returned value: \nNAVAILABLE - This feature is not available on this PNA \nReturn Type Character \nDefault At Preset: \nBNC1 = INACTIVE \nBNC2 = INACTIVE \nAUXT = TILHIGH \nWhen Output is enabled: \nBNC1 = INACTIVE \nBNC2 = TOPPAFTER \nAUXT = TILHIGH \nCONTrol:SIGNal:TRIGger:ATBA <bool> \n1583\n\n(Read-Write) Accept Trigger Before Armed Determines what happens to an EDGE trigger signal if it occurs \nbefore the PNA is ready to be triggered. (LEVEL trigger signals are always ignored.) For more information, see \nExternal triggering. \nParameters \n<bool> Boolean \nFalse (0) - A trigger signal is ignored if it occurs before the PNA is ready to be triggered. \nTrue (1) - A trigger signal is remembered and then used when the PNA becomes armed \n(ready to be triggered). The PNA remembers only one trigger signal. \nExamples CONT:SIGN:TRIG:ATBA 0 \ncontrol:signal:trigger:atba true \nQuery Syntax CONTrol:SIGNal:TRIGger:ATBA? \nReturn Type Boolean \nDefault False \nCONTrol:SIGNal:TRIGger:OUTP <bool> \n(Read-Write) Output Enabled The PNA can be enabled to send trigger signals out the rear-panel TRIGGER \nOUT BNC connector. Use CONTrol:SIGNal to configure for output triggers. \nFor more information, see External triggering. \nParameters \n<bool> Boolean \nFalse (0) - PNA does NOT output trigger signals. \nTrue (1) - PNA DOES output trigger signals. \nExamples CONT:SIGN:TRIG:OUTP 1 \ncontrol:signal:trigger:outp false \nQuery Syntax CONTrol:SIGNal:TRIGger:OUTP? \nReturn Type Boolean \nDefault False \nLast Modified: \n1584\n\n18-Jan-2007 Fixed count? example \n1585\n\nDisplay Commands \nControls the settings of the front panel screen. \n1586\n\nClick on a blue keyword to view the command details. \nSee Also \nSee an example using some of these commands \nSynchronizing the PNA and Controller \nLearn about Screen Setup \nSCPI Command Tree \nDISPlay:ANNotation:FREQuency[:STATe] <ON | OFF> \n(Read-Write) Turns frequency information on the display title bar ON or OFF for all windows. \nParameters \n<ON | OFF> ON (or 1) - turns frequency annotation ON. \nOFF (or 0) - turns frequency annotation OFF. \nExamples DISP:ANN:FREQ ON \ndisplay:annotation:frequency:state off \nQuery Syntax DISPlay:ANNotation:FREQuency[:STATe]? \nReturn Type Boolean (1 = ON, 0 = OFF) \nDefault ON (1) \nDISPlay:ANNotation:MESSage:STATe <ON | OFF> \n(Read-Write) Enables and disables error pop-up messages on the display. \nParameters \n<ON | OFF> ON (or 1) - enables error pop-up messages \nOFF (or 0) - disables error pop-up messages \nExamples DISP:ANN:MESS:STAT ON \ndisplay:annotation:message:state off \nQuery Syntax DISPlay:ANNotation:MESSage:STATe? \nReturn Type Boolean (1 = ON, 0 = OFF) \nDefault ON (1) \nDISPlay:ANNotation:STATus <ON | OFF> \n1587\n\n(Read-Write) Turns the status bar at the bottom of the screen ON or OFF. The status bar displays \ninformation for the active window. \nParameters \n<ON | OFF> ON (or 1) - turns status bar ON. \nOFF (or 0) - turns status bar OFF. \nExamples DISP:ANN:STAT ON \ndisplay:annotation:status off \nQuery Syntax DISPlay:ANNotation:STATus? \nReturn Type Boolean (1 = ON, 0 = OFF) \nDefault Last state that was set \nDISPlay:ARRange <char> \n(Write-only) Places EXISTING measurements into pre-configured window arrangements. Overlay, \nStack(2), Split(3), and Quad(4) creates new windows. To learn more, see Arrange Existing \nMeasurements. \nParameters \n<char> Window arrangement. Choose from: \nTILE - tiles existing windows \nCASCade - overlaps existing windows \nOVERlay - all traces placed in 1 window \nSTACk - 2 windows \nSPLit - 3 windows \nQUAD - 4 windows \nExamples DISP:ARR CASC \ndisplay:arrange cascade \nQuery Syntax Not Applicable \nDefault TILE \nDISPlay:CATalog? \n1588\n\n(Read-only) Returns the existing Window numbers. \nReturn Type String of Character values, separated by commas \nExample Two windows with numbers 1 and 2 returns: \n\"1,2\" \nDefault Not applicable \nDISPlay:ENABLE <ON | OFF> \n(Read-Write) Specifies whether to disable or enable all analyzer display information in all windows \nin the analyzer application. Marker data is not updated. More CPU time is spent making \nmeasurements instead of updating the display. \nParameters \n<ON | OFF> ON (or 1) - turns the display ON. \nOFF (or 0) - turns the display OFF. \nExamples DISP:ENAB ON \ndisplay:enable off \nQuery Syntax DISPlay:ENABle? \nReturn Type Boolean (1 = ON, 0 = OFF) \nDefault ON \nDISPlay:FSIGn <ON | OFF> \n(Read-Write) Shows or hides the window which displays global pass/fail results. \nParameters \n<ON | OFF> ON (or 1) - displays the pass/fail dialog \nOFF (or 0) - hides the pass/fail dialog \nExamples DISP:FSIG ON \ndisplay:fsign off \nQuery Syntax DISPlay:FSIGn? \nReturn Type Boolean (1 = ON, 0 = OFF) \nDefault OFF \nDISPlay[:TILE] - Superseded \n1589\n\nThis command is replaced by DISP:ARRange \n(Write-only) Tiles the windows on the screen. \nExamples DISP \ndisplay:tile \nDefault Not Applicable \nDISPlay:WINDow<wnum>:ANNotation:MARKer:SINGle[:STATe] <bool> \n(Read-Write) Either shows marker readout of only the active trace or other traces simultaneously. \nSee other SCPI Marker commands. Learn more about Marker readout. \nParameters \n<wnum> Any existing window number. If unspecified, value is set to 1. \n<bool> ON (or 1) - Shows the readout of only the active marker for each trace. \nOFF (or 0) - Shows up to 5 marker readouts per trace, up to 20 total readouts. \nExamples DISP:WIND:ANN:MARK:SING ON \ndisplay:window:annotation:marker:single off \nQuery Syntax DISPlay:WINDow:ANNotation:MARKer:SINGle? \nReturn Type Boolean (1 = ON, 0 = OFF) \nDefault OFF \nDISPlay:WINDow<wnum>:ANNotation:MARKer:SIZE <char> \n(Read-Write) Specifies the size of the marker readout text. See other SCPI Marker commands. Learn \nmore about Marker readout. \nParameters \n<wnum> Any existing window number. If unspecified, value is set to 1. \n<char> Readout text size. Choose from:NORMal | LARGe \nExamples DISP:WIND:ANN:MARK:SIZE LARG \ndisplay:window:annotation:marker:size normal \nQuery Syntax DISPlay:WINDow:ANNotation:MARKer:SIZE? \nReturn Type Character \nDefault NORMal \n1590\n\nDISPlay:WINDow<wnum>:ANNotation:MARKer:STATe <ON | OFF> \n(Read-Write) Specifies whether to show or hide the Marker readout (when markers are ON) on the \nselected window. See other SCPI Marker commands. Learn more about Marker readout. \nParameters \n<wnum> Any existing window number. If unspecified, value is set to 1. \n<ON | OFF> ON (or 1) - turns marker readout ON. \nOFF (or 0) - turns marker readout OFF. \nExamples DISP:WIND:ANN:MARK:STAT ON \ndisplay:window:annotation:marker:state off \nQuery Syntax DISPlay:WINDow:ANNotation:MARKer:STATe? \nReturn Type Boolean (1 = ON, 0 = OFF) \nDefault ON \nDISPlay:WINDow<wnum>:ANNotation:TRACe:STATe <ON | OFF> \n(Read-Write) Specifies whether to show or hide the Trace Status buttons on the left of the display. \nParameters \n<wnum> Any existing window number. If unspecified, value is set to 1. \n<ON | OFF> ON (or 1) - turns the buttons ON. \nOFF (or 0) - turns the buttons OFF. \nExamples DISP:WIND:ANN:TRAC:STAT ON \ndisplay:window:annotation:trace:state off \nQuery Syntax DISPlay:WINDow:ANNotation:TRACe:STATe? \nReturn Type Boolean (1 = ON, 0 = OFF) \nDefault ON \nDISPlay:WINDow<wnum>:CATalog? \n1591\n\n(Read-only) Returns the trace numbers for the specified window. \nParameters \n<wnum> Any existing window number. If unspecified, value is set to 1. \nExample Window 1 with four traces: \nDISPlay:WINDow1:CATalog? \nReturns: \n\"1,2,3,4\" \nReturn Type String of Character values separated by commas \nDefault Not applicable \nDISPlay:WINDow<wnum>:ENABle <ON | OFF> \n(Read-Write) Specifies whether to disable or enable all analyzer display information in the specified \nwindow. Marker data is not updated. More CPU time is spent making measurements instead of \nupdating the display. \nParameters \n<wnum> Any existing window number. If unspecified, value is set to 1. \n<ON | OFF> ON (or 1) - turns the display ON. \nOFF (or 0) - turns the display OFF. \nExamples DISP:WIND:ENABle ON \ndisplay:window1:enable off \nQuery Syntax DISPlay:WINDow<wnum>:ENABle? \nReturn Type Boolean (1 = ON, 0 = OFF) \nDefault ON \nDISPlay:WINDow<wnum>:SIZE <char> \n1592\n\n(Read-Write) Sets or returns the window setting of Maximized, Minimized, or Normal. To arrange all \nof the windows, use DISP:ARR. \nParameters \n<wnum> Any existing window number. If unspecified, value is set to 1 \n<char> Window size. Choose from: \nMIN | MAX | NORM \nExamples DISP:WIND:SIZE MAX \ndisplay:window:size norm \nQuery Syntax DISPlay:WINDow:SIZE? \nDefault Not Applicable \nDISPlay:WINDow<wnum>[:STATe] <ON | OFF> \n(Read-Write) Write to create or delete a window on the screen or Read whether a window is present. \nParameters \n<wnum> Window number to create; choose any integer between 1 and the maximum \nnumber of windows allowed in the PNA. \n<ON | OFF> ON (or 1) - The window <wnum> is created. \nOFF (or 0) - The window <wnum> is deleted. \nExamples DISP:WIND ON \ndisplay:window2:state off \nQuery Syntax DISPlay:WINDow<wnum>[:STATe]? \nReturn Type Boolean (1 = ON, 0 = OFF) \nDefault Window number \"1\" ON \nDISPlay:WINDow<wnum>:TABLe <char> \n1593\n\n(Read-Write) Write to show the specified table at the bottom of the analyzer screen or Read to \ndetermine what table is visible. \nParameters \n<wnum> Any existing window number. If unspecified, value is set to 1 \n<char> Table to show. Choose from: \nOFF | MARKer | LIMit | SEGMent \nExamples DISP:WIND:TABLe SEGM \ndisplay:window:table off \nQuery Syntax DISPlay:WINDow:TABLe? \nDefault OFF \nDISPlay:WINDow<wnum>:TITLe:DATA <string> \n(Read-Write) Sets data in the window title area. The title is turned ON and OFF with \nDISP:WIND:TITL:STAT OFF. \nParameters \n<wnum> Any existing window number. If unspecified, value is set to 1. \n<string> Title to be displayed. Any characters, enclosed with quotes. If the title string \nexceeds 50 characters, an error will be generated and the title not accepted. \nNewer entries replace (not append) older entries. \nExamples DISP:WIND:TITL:DATA 'hello' \ndisplay:window2:title:data 'hello' \nQuery Syntax DISPlay:WINDow<wnum>:TITLe:DATA? \nReturn Type String \nDefault NA \nDISPlay:WINDow<wnum>:TITLe[:STATe] <ON | OFF> \n1594\n\n(Read-Write) Turns display of the title string ON or OFF. When OFF, the string remains, ready to be \nredisplayed when turned back ON. \nParameters \n<wnum> Any existing window number. If unspecified, value is set to 1 \n<ON | OFF> ON (or 1) - turns the title string ON. \nOFF (or 0) - turns the title string OFF. \nExamples DISP:WIND:TITL ON \nDisplay:window1:title:state off \nQuery Syntax DISPlay:WINDow<wnum>:TITLe[:STATe]? \nReturn Type Boolean (1 = ON, 0 = OFF) \nDefault ON \nDISPlay:WINDow<wnum>:TRACe<tnum>:DELete \n(Write-only) Deletes the specified trace from the specified window. The measurement parameter \nassociated with the trace is not deleted. \nParameters \n<wnum> Any existing window number. If unspecified, value is set to 1. \n<tnum> The number of the trace to be deleted; if unspecified, value is set to 1 \nExamples DISP:WIND:TRAC:DEL \ndisplay:window2:trace2:delete \nQuery Syntax Not applicable \nDefault NA \nDISPlay:WINDow<wnum>:TRACe<tnum>:FEED <name> \n1595\n\n(Write-only) Creates a new trace <tnum> and associates (feeds) a measurement <name> to the \nspecified window<wnum>. This command should be executed immediately after creating a new \nmeasurement with CALC:PAR:DEF<name>,<parameter>. \nTo feed the same measurement to multiple traces, create another measurement with the same \n<name>,<parameter> using the CALC:PAR:DEF command. The analyzer will collect the data only \nonce. \nParameters \n<wnum> Any existing window number. If unspecified, value is set to 1. \n<tnum> Trace number to be created. Choose any Integer between 1 and 8 \n<name> Name of the measurement that was defined with \nCALC:PAR:DEF<name>,<parameter> \nExamples DISP:WIND:TRAC:FEED 'test' \ndisplay:window2:trace2:feed 'test' \nQuery Syntax Not applicable \nDefault \"CH1_S11\" \nDISPlay:WINDow<wnum>:TRACe<tnum>MEMory[:STATe] <ON | OFF> \n(Read-Write) Turns the memory trace ON or OFF. \nParameters \n<wnum> Any existing window number. If unspecified, value is set to 1. \n<tnum> Any existing trace number; if unspecified, value is set to 1 \n<ON | OFF> ON (or 1) - turns the memory trace ON. \nOFF (or 0) - turns the memory trace OFF. \nExamples DISP:WIND:TRAC:MEM ON \ndisplay:window2:trace2:memory:state off \nQuery Syntax DISPlay:WIND<wnum>:TRACe<tnum>:MEMory[:STATe]? \nReturn Type Boolean (1 = ON, 0 = OFF) \nDefault OFF \nDISPlay:WINDow<wnum>:TRACe<tnum>:SELect \n1596\n\n(Write-only) Activates the specified trace in the specified window for front panel use. \nParameters \n<wnum> Any existing window number. If unspecified, value is set to 1. \n<tnum> Any existing trace number; if unspecified, value is set to 1 \nExamples DISP:WIND:TRAC:SEL \ndisplay:window2:trace2:select \nQuery Syntax Not applicable \nDefault NA \nDISPlay:WINDow<wnum>:TRACe<tnum>[:STATe] <ON | OFF> \n(Read-Write) Turns the display of the specified trace in the specified window ON or OFF. When OFF, \nthe measurement behind the trace is still active. \nParameters \n<wnum> Any existing window number. If unspecified, value is set to 1. \n<tnum> Any existing trace number; if unspecified, value is set to 1 \n<ON | OFF> ON (or 1) - turns the trace ON. \nOFF (or 0) - turns the trace OFF. \nExamples DISP:WIND:TRAC ON \ndisplay:window2:trace2:state off \nQuery Syntax DISPlay:WIND<wnum>:TRACe<tnum>[:STATe]? \nReturn Type Boolean (1 = ON, 0 = OFF) \nDefault ON \nDISPlay:WINDow<wnum>:TRACe<tnum>TITLe:DATA <string> \n1597\n\n(Read-Write) Writes and read data to the trace title area. The trace title is embedded in the trace status \nfield. Learn more. \nNewer entries replace (not append) older entries. The title is turned ON and OFF with \nDISP:WIND:TRAC:TITL:STAT. \nParameters \n<wnum> Any existing window number. If unspecified, value is set to 1. \n<tnum> Trace number of the specified window. If unspecified, value is set to 1. The \ntrace number displayed in trace status is the trace number of the channel; not \nthe window. Use Display:Cat? to read the window numbers. Use \nDisp:Window:Cat? to read the trace numbers of the specified window. \n<string> Title to be displayed. Any characters (not spaces) enclosed with quotes. \nExamples DISP:WIND:TRAC:TITL:DATA 'MyNewMeas' \ndisplay:window2:trace3:title:data 'hello' \nQuery Syntax 
